vi "p8.3.vi"() -> ()   [LabVIEW 2020]
uses:
  <vilib>/vision/NI_Vision_Development_Module.lvlib
panel:
  in  "Tipo imagen2":T1=1 items=["Grayscale (U8)", "Grayscale (I16)", "Grayscale (SGL)", "Complex (CSG)", "RGB (U32)", "HSL (U32)", "RGB (U64)", "Grayscale (U16)"]
  in  "Tipo imagen1":T1=1 items=["Grayscale (U8)", "Grayscale (I16)", "Grayscale (SGL)", "Complex (CSG)", "RGB (U32)", "HSL (U32)", "RGB (U64)", "Grayscale (U16)"]
  out "Histograma Imagen_suma":T2(graph)={"Starting Value"=0.0, "Incremental Value"=1.0, "Histogram"=[3831, 310, 229, 65, 49, 41, 31, 46, 35, 20, 22, 15, 13, 12, 19, 1, 7, 3, 7, 4, 1, 8, 7, 2, 6, 8, 4, 5, 18, 13, 7, 14, 12, 9, 7, 15, 6, 7, 10, 13, 7, 11, 9, 12, 15, 14, 13, 16, 9, 12, 7, 23, 11, 13, 17, 20, 19, 18, 17, 14, 10, 10, 11, 13, 15, 13, 14, 11, 6, 4, 5, 9, 7, 6, 12, 11, 7, 9, 12, 13, 22, 13, 19, 22, 22, 25, 15, 32, 43, 41, 40, 25, 25, 27, 42, 28, 46, 36, 46, 48, 48, 39, 42, 40, 40, 30, 29, 44, 37, 19, 34, 28, 23, 25, 35, 21, 23, 22, 20, 15, 14, 22, 22, 22, 24, 30, 24, 23, 21, 18, 14, 25, 22, 25, 25, 31, 45, 26, 22, 35, 24, 26, 30, 41, 29, 22, 39, 39, 40, 41, 44, 44, 51, 58, 48, 52, 44, 43, 50, 37, 40, 51, 36, 38, 48, 43, 40, 46, 27, 44, 46, 35, 37, 46, 44, 49, 69, 61, 72, 51, 61, 60, 61, 61, 73, 61, 66, 56, 52, 59, 70, 58, 71, 67, 44, 66, 67, 62, 60, 67, 58, 63, 52, 53, 46, 40, 42, 53, 36, 42, 41, 45, 36, 52, 42, 43, 48, 21, 49, 37, 35, 42, 27, 34, 31, 59, 58, 69, 72, 59, 62, 53, 71, 62, 41, 47, 55, 57, 58, 46, 37, 43, 57, 68, 54, 63, 42, 43, 33, 36, 24, 25, 23, 20, 23, 12977]}
  out "Imagen_suma":T3(plugin-control)
  out "Imagen2":T3(plugin-control)
  out "Imagen1":T3(plugin-control)
  in  "Path imagen2":path=path "Z:/BenoBelmont/teleco2020_21/TDS/laboratorio/P789/imagenes_monocromas/160_160/escalagrises_mono.tif"
  in  "Path imagen1":path=path "Z:/BenoBelmont/teleco2020_21/TDS/laboratorio/P789/imagenes_monocromas/160_160/ajedrez_mono.tif"
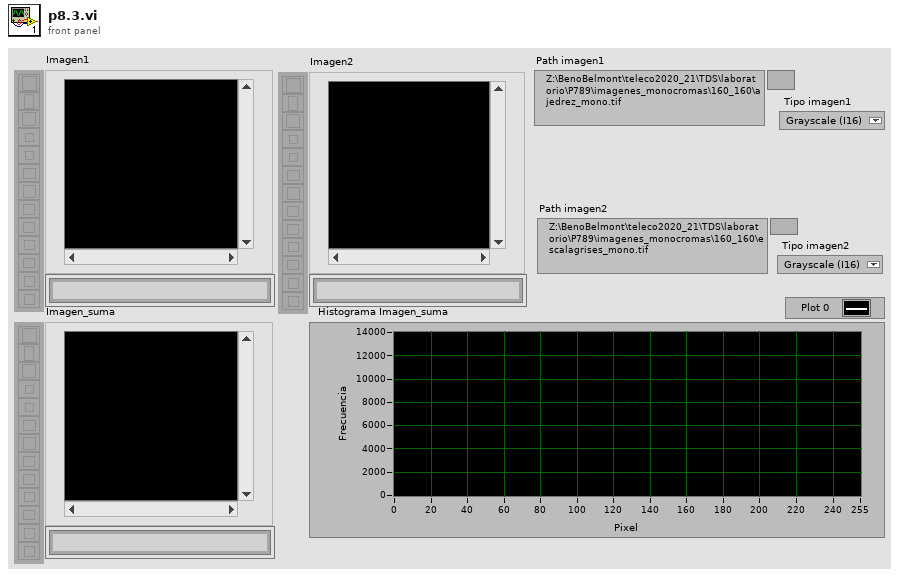
[diagram p1: front panel]
types:
  T1 = typedef "Image Type" = u32
  T2 = cluster{"Starting Value":sgl, "Incremental Value":sgl, "Histogram":u32[]}
  T3 = typedef "IMAQ Image.ctl" = refnum<image>
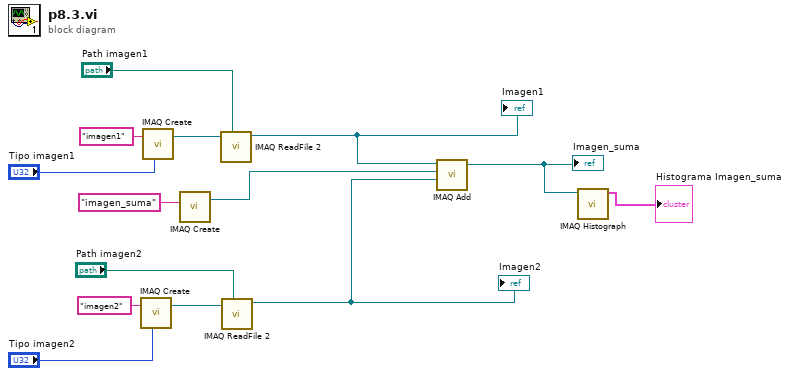
[diagram p0: block diagram]
diagram:
  n1 = call "IMAQ Create"("Image Name"="imagen2", "Image Type"="Tipo imagen2") -> ("New Image"=w10:T3)  [unwired: 3 in, 1 out]
  n2 = call "IMAQ Create"("Image Name"="imagen1", "Image Type"="Tipo imagen1") -> ("New Image"=w11:T3)  [unwired: 3 in, 1 out]
  n3 = call "IMAQ Create"("Image Name"="imagen_suma") -> ("New Image"=w5:T3)  [unwired: 4 in, 1 out]
  n4 = call "IMAQ ReadFile 2"("File Path"="Path imagen1", "Image"=w11) -> ("Image Out"=w8:T3)  [unwired: 5 in, 4 out]
  "Imagen1" <- w8
  n5 = call "IMAQ ReadFile 2"("File Path"="Path imagen2", "Image"=w10) -> ("Image Out"=w7:T3)  [unwired: 5 in, 4 out]
  "Imagen2" <- w7
  n6 = call "IMAQ Add"("Image Src A"=w8, "Image Dst"=w5, "Image Src B"=w7) -> ("Image Dst Out"=w4:T3)  [unwired: 4 in, 1 out]
  "Imagen_suma" <- w4
  n7 = call "IMAQ Histograph"("Image"=w4) -> ("Histogram Graph"=→"Histograma Imagen_suma":T2)  [unwired: 7 in, 3 out]
